vi "RunConstantImageStimulus.vi"() -> ()   [LabVIEW 2019]
uses:
  Parameters.ctl
  ConstantImageStimulusClass/ConstantImageStimulus.lvclass
  C:/Users/mochil/Dropbox/LeiferShaevitz/Github/ProjectAPI/LabviewVIs/StimulusObject.lvclass
panel:
  out "selected path":path
  out "error IO":errorcluster
  in  "Start":bool
  in  "Wait Before Recording (s)":u32
  in  "SSH password":string
  in  "SSH user name":string
  in  "Last Experiment of the Day":bool
  in  "Tags":string
  out "Parameters":T1 {"FW_WormLengthSD" format="%#.6e"}
  # "Faux Worm Drawing"
  # "Tracking"
  # "Temporal Calibration"
  # "Stimulus Generation"
  # "Median Filtering"
  # "Experimental Settings"
  # "Camera and Projector Settings"
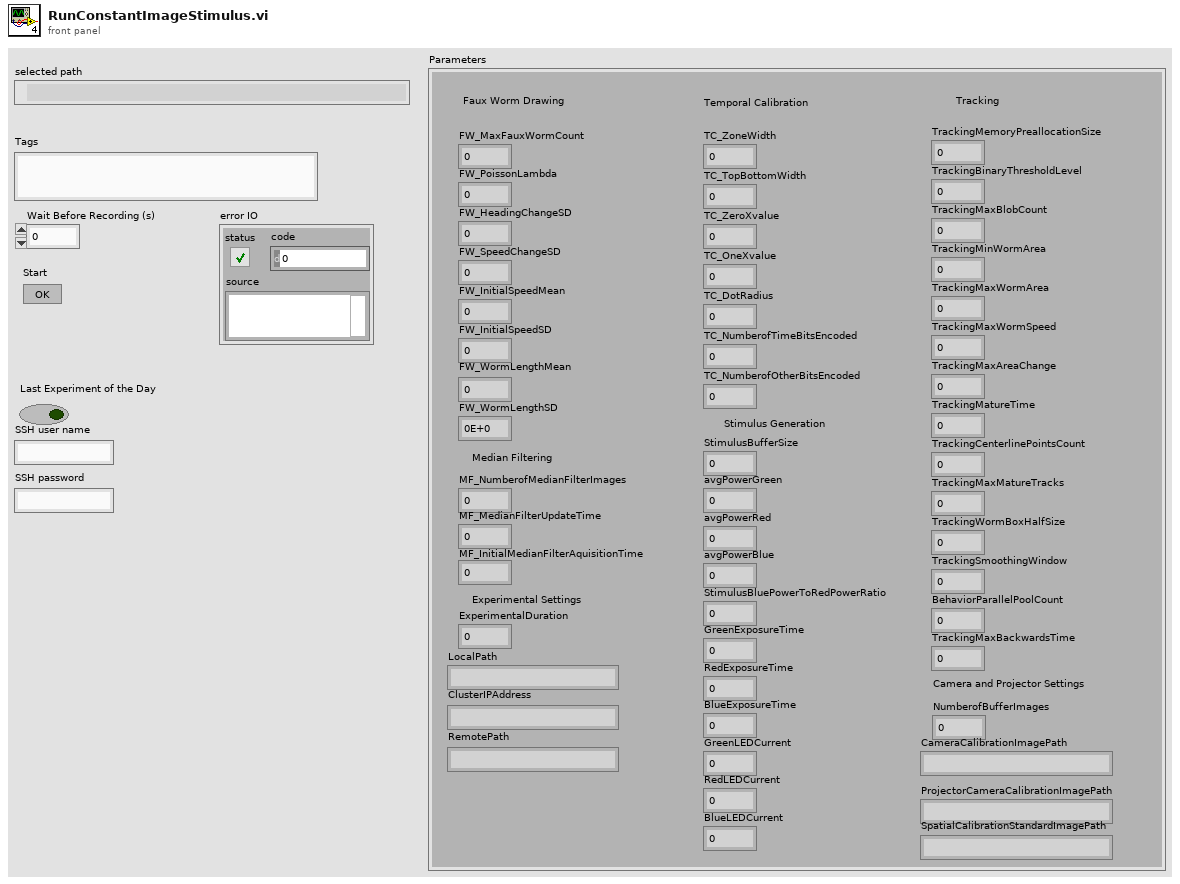
[diagram p1: front panel]
types:
  T1 = typedef "Parameters.ctl" = cluster{"FW_MaxFauxWormCount":i32, "FW_PoissonLambda":dbl, "FW_HeadingChangeSD":dbl, "FW_SpeedChangeSD":dbl, "FW_InitialSpeedMean":dbl, "FW_InitialSpeedSD":dbl, "FW_WormLengthMean":dbl, "FW_WormLengthSD":dbl, "MF_NumberofMedianFilterImages":i32, "MF_MedianFilterUpdateTime":i32, "MF_InitialMedianFilterAquisitionTime":dbl, "ExperimentalDuration":i32, "TC_ZoneWidth":i32, "TC_TopBottomWidth":i32, "TC_ZeroXvalue":i32, "TC_OneXvalue":i32, "TC_DotRadius":i32, "TC_NumberofTimeBitsEncoded":i32, "TC_NumberofOtherBitsEncoded":i32, "NumberofBufferImages":sgl, "CameraCalibrationImagePath":string, "ProjectorCameraCalibrationImagePath":string, "StimulusBufferSize":i32, "TrackingMemoryPreallocationSize":i32, "TrackingBinaryThresholdLevel":sgl, "TrackingMaxBlobCount":i32, "TrackingMinWormArea":dbl, "TrackingMaxWormArea":dbl, "TrackingMaxWormSpeed":dbl, "TrackingMaxAreaChange":dbl, "TrackingMatureTime":i32, "TrackingCenterlinePointsCount":i32, "TrackingMaxMatureTracks":i32, "TrackingWormBoxHalfSize":i32, "TrackingSmoothingWindow":i32, "BehaviorParallelPoolCount":i32, "LocalPath":string, "GreenExposureTime":i32, "RedExposureTime":i32, "BlueExposureTime":i32, "ClusterIPAddress":string, "RemotePath":string, "GreenLEDCurrent":u8, "RedLEDCurrent":u8, "BlueLEDCurrent":u8, "avgPowerGreen":sgl, "avgPowerRed":sgl, "avgPowerBlue":sgl, "StimulusBluePowerToRedPowerRatio":sgl, "SpatialCalibrationStandardImagePath":string, "TrackingMaxBackwardsTime":i32}
  T2 = typedef "Image Type" = u32
  T3 = typedef "IMAQ Image.ctl" = refnum<image>
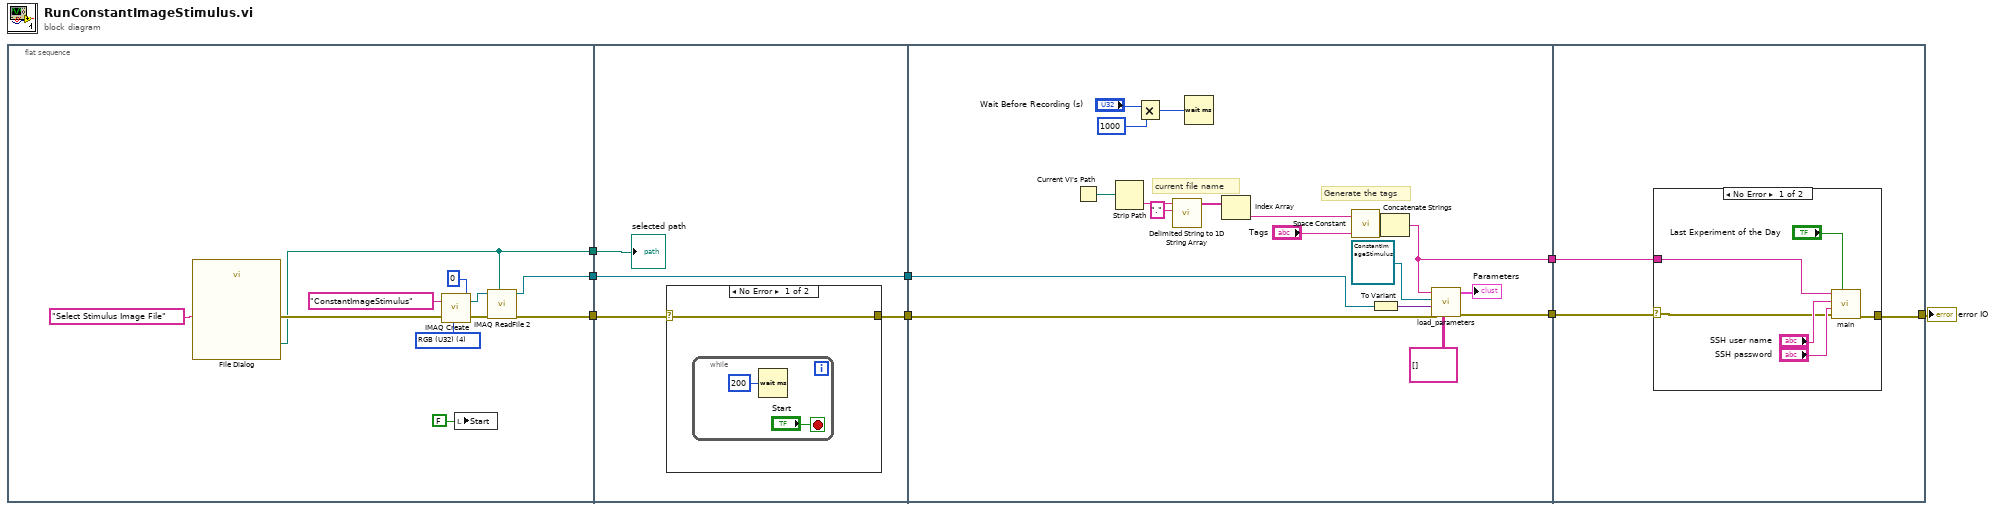
[diagram p0: block diagram]
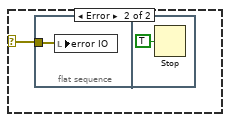
[diagram p2: hidden frame]
diagram:
  n1 = flat-sequence {
    tunnel: [w12] -> w5
    tunnel: [w10] -> w2
    tunnel: [w9] -> w1
    tunnel: w5 -> [w23]
    tunnel: [w22] -> w4
    tunnel: [w21] -> w3
    tunnel: w2 -> [w21]
    tunnel: w1 -> [w20]
    tunnel: [w47] -> w8
    tunnel: [w43] -> w7
    tunnel: w4 -> [w32]
    tunnel: w3 -> [w31]
    tunnel: w7 -> [w49]
    tunnel: w8 -> [w50]
    tunnel: [w48] -> w6
    frame #0 {
      w13 = T2 4 items=["Grayscale (U8)", "Grayscale (I16)", "Grayscale (SGL)", "Complex (CSG)", "RGB (U32)", "HSL (U32)", "RGB (U64)", "Grayscale (U16)"] ("Image Type")
      n2 = call "File Dialog"("prompt"="Select Stimulus Image File") -> ("selected path"=w9:path, "error out"=w16:errorcluster)  [unwired: 11 in, 2 out]
      n3 = call "IMAQ Create"("Border Size"=0, "Image Name"="ConstantImageStimulus", "Image Type"=w13, "error in (no error)"=w16) -> ("New Image"=w18:T3, "error out"=w17:errorcluster)  [unwired: 1 in]
      n4 = local write "Start"(FALSE ("Start")) -> ()
      n5 = call "IMAQ ReadFile 2"("File Path"=w9, "error in (no error)"=w17, "Image"=w18) -> ("error out"=w12:errorcluster, "Image Out"=w10:T3)  [unwired: 4 in, 3 out]
    }
    frame #1 {
      n6 = case shown="No Error" w23 {
        selector: w23 -> [w24 w27]
        tunnel: [w24 _] -> w22
        frame No Error {
          n7 = while {
            stop <- "Start" stop-if-true
            n8 = Wait (ms)(milliseconds to wait=u32 200) -> ()  [unwired: 1 out]
          }
        }
        frame Error {
          n9 = flat-sequence {
            tunnel: w27 -> [w28]
            frame #0 {
              n10 = local write "error IO"(w28) -> ()
            }
            frame #1 {
              n11 = Stop(stop? (T)=TRUE) -> ()
            }
          }
        }
      }
      "selected path" <- w20
    }
    frame #2 {
      # "current file name"
      # "Generate the tags"
      n12 = Current VI's Path() -> (path=w39:path)
      n13 = Strip Path(path=w39) -> (name=w38:string)  [unwired: 1 out]
      n14 = Multiply(x="Wait Before Recording (s)", y=u32 1000) -> (x*y=w40:u32)
      n15 = call <vilib>:"Delimited String to 1D String Array.vi"("delimiter"=".", "delimited string"=w38) -> ("string array"=w36:string[])  [unwired: 9 in]
      n16 = Wait (ms)(milliseconds to wait=w40) -> ()  [unwired: 1 out]
      n17 = Index Array(array=w36) -> (element=w35:string)  [unwired: 1 in]
      n18 = call <vilib>:"Space Constant.vi"() -> ("String"=w44:string)
      n19 = To Variant(anything=w31) -> (Variant=w30:variant)
      n20 = Concatenate Strings(w35, w44, "Tags") -> (w43:string)
      n21 = call "load_parameters.vi"("additional loaded parameters to write"=string[][] [], "error in (no error)"=w32, "StimulusObject Parameters"=w30, "StimulusObjectClassInput"=refnum<class "ConstantImageStimulus.lvclass"> refnum ("ConstantImageStimulus.lvclass"), "Tags"=w43) -> ("error out"=w47:errorcluster, "Parameters"=→"Parameters":T1)  [unwired: 4 in, 1 out]
    }
    frame #3 {
      n22 = case shown="No Error" w50 {
        selector: w50 -> [w53 w57]
        tunnel: [w52 w57] -> w48
        tunnel: w49 -> [w51 _]
        frame No Error {
          n23 = call "main.vi"("Last Experiment of the Day"="Last Experiment of the Day", "error in"=w53, "SSH password"="SSH password", "SSH user name"="SSH user name", "Tags"=w51) -> ("error out"=w52:errorcluster)  [unwired: 6 in]
        }
        frame Error {
        }
      }
    }
  }
  "error IO" <- w6
